vi "AddOffsetToWaveform.vi"(0 "Waveform In":waveform(dbl)={"t0"=timestamp(3433165898.5470004 s since 1904-01-01), "dt"=1e-05, "Y"=array[4250 elements]}, 9 "Offset":dbl=1.0) -> (4 "Waveform out":waveform(dbl)={"t0"=timestamp(3433165898.5470004 s since 1904-01-01), "dt"=1e-05, "Y"=array[4250 elements]})   [LabVIEW 2010]
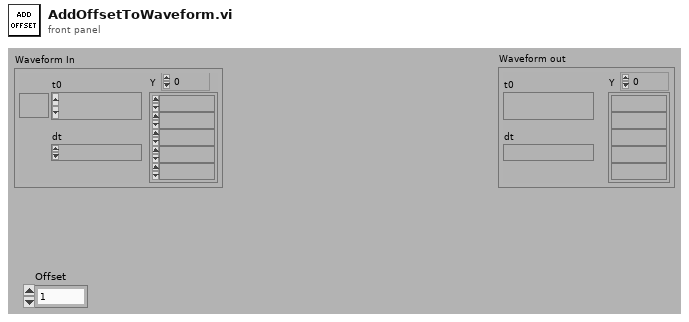
[diagram p1: front panel]
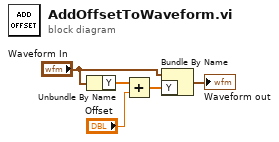
[diagram p0: block diagram]
diagram:
  n1 = Unbundle By Name("Waveform In") -> ("Y"=w5:dbl[])
  n2 = Add(x=w5, y="Offset") -> (x+y=w2:dbl[])
  n3 = Bundle By Name(cluster="Waveform In", "Y"=w2) -> (→"Waveform out":waveform(dbl))
